vi "Generate Payload.vi"(9 "PRBS degree":T1 items=["7", "9", "10", "11", "15", "17", "18", "20", "21", "22", "23", "25"], 10 "payload length":i32, 11 "preamble symbol":i32) -> (3 "bit stream":bool[](array[boolean]))   [LabVIEW 2025, in "SOQPSK Host Support.lvlib"]
uses:
  SOQPSK Host Support.lvlib
  Program Files/NI/LVAddons/dltf/1/examples/Data Link Test Framework/Modems/Shared/BER/FPGA/PRBS/PRBS Degree Selection.ctl
  Program Files/NI/LVAddons/dltf/1/examples/Data Link Test Framework/Modems/Shared/BER/Host/BER Host.lvclass
  Program Files/NI/LVAddons/dltf/1/examples/Data Link Test Framework/Modems/Shared/BER/FPGA/PRBS/PRBS.lvlib
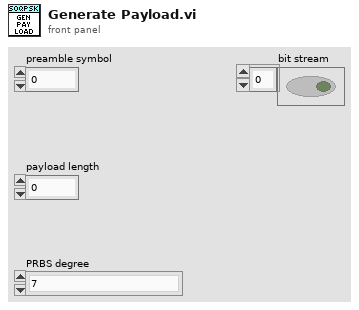
[diagram p1: front panel]
types:
  T1 = typedef "Modems Shared.lvlib/PRBS.lvlib/PRBS Degree Selection.ctl" = u16
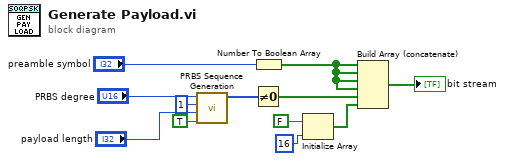
[diagram p0: block diagram]
diagram:
  n1 = call "PRBS Sequence Generation.vi"("backward"=TRUE, "total bits"="payload length", "seed"=u32 1, "PRBS degree"="PRBS degree") -> ("bit stream"=w2:i16[])  [unwired: 6 in, 1 out]
  n2 = Not Equal To 0?(x=w2) -> (x != 0?=w1:bool[])
  n3 = Number To Boolean Array(number="preamble symbol") -> (Boolean array=w8:bool[])
  n4 = Initialize Array(FALSE, 16 ("dimension size")) -> (w12:bool[])
  n5 = Build Array (concatenate)(w8, w8, w8, w8, w1, w12) -> (→"bit stream":bool[])
